vi "rad_hms.vi"(3 "TRUE=HORA\nFALSE=GRAU":bool, 5 "Radiano":dbl format="%#.18g") -> (2 "Hora/Graus Texto Decimal":string)   [LabVIEW 2012]
panel:
  in  "Case Constant\n(See Context Help)":bool
  out "Segundos":string
  out "Minutos":string
  out "Graus":string
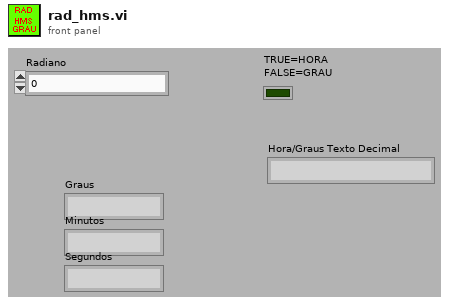
[diagram p1: front panel]
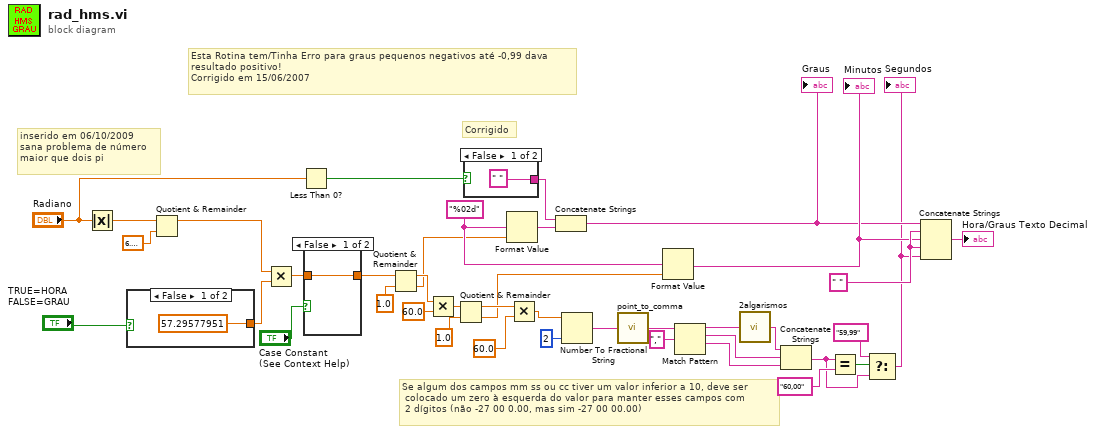
[diagram p0: block diagram]
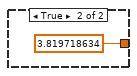
[diagram p2: hidden frame]
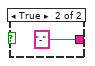
[diagram p3: hidden frame]
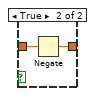
[diagram p4: hidden frame]
diagram:
  w30 = "%02d" ("format string")
  w34 = " "
  # "inserido em 06/10/2009\nsana problema de número\nmaior que dois pi"
  # "Se algum dos campos mm ss ou cc tiver um valor inferior a 10, deve ser\n colocado um zero à esquerda do valor para manter esses campos com\n 2 dígitos (não -27 00 0.00, mas sim -27 00 00.00)"
  # "Corrigido"
  # "Esta Rotina tem/Tinha Erro para graus pequenos negativos até -0,99 dava\nresultado positivo!\nCorrigido em 15/06/2007"
  n1 = Absolute Value(x="Radiano") -> (abs(x)=w1:dbl)
  n2 = case shown="False" "TRUE=HORA\nFALSE=GRAU" {
    tunnel: [57.29577951 ("x*y") 3.819718634 ("x*y")] -> w17
    frame False {
    }
    frame True {
    }
  }
  n3 = Quotient & Remainder(x=w1, y=6.283185307179586) -> (x-y*floor(x/y)=w13:dbl)  [unwired: 1 out]
  n4 = Multiply(x=w13, y=w17) -> (x*y=w19:dbl)
  n5 = Less Than 0?(x="Radiano") -> (x < 0?=w11:bool)
  n6 = case shown="False" "Case Constant\n(See Context Help)" {
    tunnel: w19 -> [w43 w44]
    tunnel: [w43 w45] -> w32
    frame False {
    }
    frame True {
      n7 = Negate(x=w44) -> (-x=w45:dbl)
    }
  }
  n8 = Quotient & Remainder(x=w32, y=1.0) -> (x-y*floor(x/y)=w36:dbl, floor(x/y)=w29:dbl)
  n9 = Multiply(x=w36, y=60.0) -> (x*y=w38:dbl)
  n10 = Quotient & Remainder(x=w38, y=1.0) -> (x-y*floor(x/y)=w40:dbl, floor(x/y)=w31:dbl)
  n11 = case shown="False" w11 {
    tunnel: [" " "-"] -> w10
    frame False {
    }
    frame True {
    }
  }
  n12 = Format Value(format string=w30, value (0)=w29) -> (output string=w15:string)  [unwired: 1 in]
  n13 = Multiply(x=w40, y=60.0) -> (x*y=w7:dbl)
  n14 = Concatenate Strings(w10, w15) -> (w16:string)
  "Graus" <- w16
  n15 = Number To Fractional String(number=w7, precision (6)=i16 2) -> (F-format string=w27:string)  [unwired: 2 in]
  n16 = call "point_to_comma.vi"("Lat_A"=w27) -> ("Saída"=w25:string)
  n17 = Format Value(format string=w30, value (0)=w31) -> (output string=w28:string)  [unwired: 1 in]
  "Minutos" <- w28
  n18 = Match Pattern(string=w25, regular expression=",") -> (before substring=w23:string, match substring=w21:string, after substring=w20:string)  [unwired: 1 in, 1 out]
  n19 = call "2algarismos.vi"("entrada"=w23) -> ("saida"=w22:string)
  n20 = Concatenate Strings(w22, w21, w20) -> (w4:string)
  n21 = Equal?(x=w4, y="60,00") -> (x = y?=w5:bool)
  n22 = Select(t="59,99" ("y"), s=w5, f=w4) -> (s? t:f=w2:string)
  "Segundos" <- w2
  n23 = Concatenate Strings(w16, w34, w28, w34, w2) -> (→"Hora/Graus Texto Decimal":string)
